vi "test Acyclic Loopback Selective Triggers.vi"(8 "error in":errorcluster, 11 "TestCase in":refnum<class "Single Board Loopback.lvclass">) -> (0 "error out":errorcluster, 3 "TestCase out":refnum<class "Single Board Loopback.lvclass">)   [LabVIEW 2020, in "Single Board Loopback.lvclass"]
uses:
  Single Board Loopback.lvclass
  C:/dev/git/niveristand-custom-device-testing-tools/VeriStandTestCase/VeriStandTestCase.lvclass
  <vilib>/numeric/Random Number (Range) U64.vi
  <vilib>/numeric/sub_Random U32.vi
  <vilib>/NI VeriStand/Execution/Workspace/NI VeriStand - Set Multiple Channel Values.vi
  <vilib>/addons/_JKI Toolkits/VI Tester/TestCase.llb/TestCase.lvclass
  <vilib>/NI VeriStand/Execution/Workspace/NI_VS Workspace ExecutionAPI.lvlib
  niveristand-custom-device-testing-tools/VeriStandTestUtilities/VeriStandTestUtilities.lvlib
  C:/Program Files (x86)/National Instruments/LabVIEW 2020/vi.lib/addons/_JKI Toolkits/VI Tester/TestCase.llb/TestCase.lvclass
  C:/dev/git/niveristand-aim-arinc429-custom-device/Source/Custom Device Support/Tests/System/Single Board Loopback/Single Board Loopback.lvclass
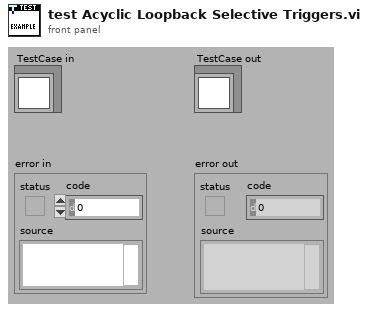
[diagram p1: front panel]
types:
  T1 = typedef "NI_VS Workspace ExecutionAPI.lvlib/WorkspaceAPI.ctl" = refnum<k24>
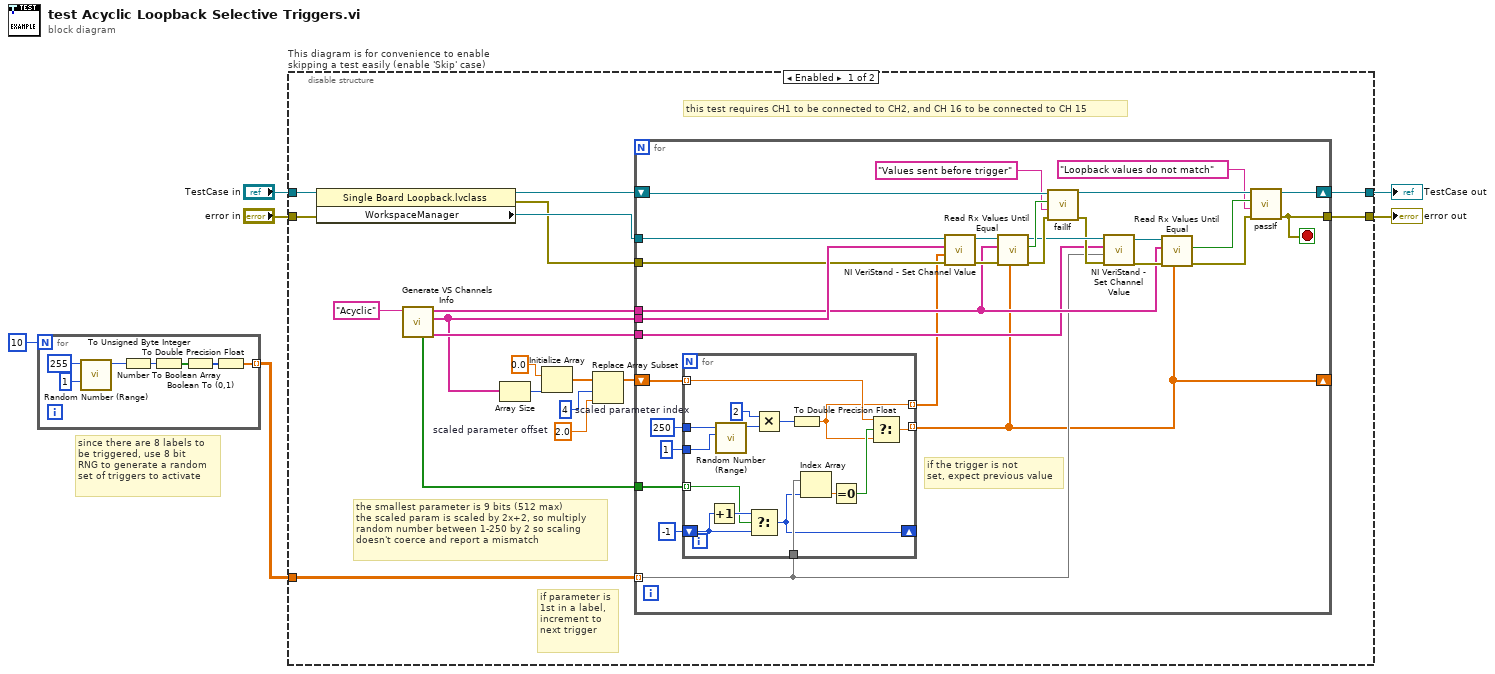
[diagram p0: block diagram]
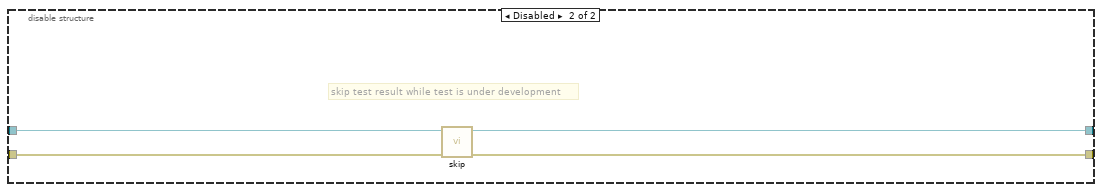
[diagram p2: hidden frame]
diagram:
  # "since there are 8 labels to\nbe triggered, use 8 bit \nRNG to generate a random\nset of triggers to activate"
  n1 = for {
    N: 10 -> [_]
    tunnel: [w7] -> w2 mode=indexing
    n2 = call-poly <vilib>:"Random Number (Range).vi"("lower bound (0)"=u64 1, "upper bound (100)"=u64 255) -> ("number"=w10:u64)  [unwired: 9 in]
    n3 = To Unsigned Byte Integer(number=w10) -> (unsigned 8bit integer=w9:u8)
    n4 = Number To Boolean Array(number=w9) -> (Boolean array=w13:bool[])
    n5 = Boolean To (0,1)(Boolean=w13) -> (0, 1=w8:i16[])
    n6 = To Double Precision Float(number=w8) -> (double precision float=w7:dbl[])
  }
  n7 = disable-structure "This diagram is for convenience to enable skipping a test easily (enable 'Skip' case)" shown="Enabled" {
    disable-tunnel: "TestCase in" -> [w28 w80]
    disable-tunnel: [w26 w78] -> w3
    disable-tunnel: [w25 w79] -> w5
    disable-tunnel: "error in" -> [w27 w77]
    disable-tunnel: w2 -> [w23 _]
    frame Enabled {
      w17 = 2.0  # scaled parameter offset
      w18 = 4  # scaled parameter index
      # "the smallest parameter is 9 bits (512 max)\nthe scaled param is scaled by 2x+2, so multiply \nrandom number between 1-250 by 2 so scaling\ndoesn't coerce and report a mismatch"
      # "if parameter is 1st in a label, increment to next trigger"
      # "this test requires CH1 to be connected to CH2, and CH 16 to be connected to CH 15"
      n8 = property class="Single Board Loopback.lvclass"(reference=w28, error in=w27) -> (reference out=w29:refnum<class "Single Board Loopback.lvclass">, error out=w30:errorcluster, "WorkspaceManager"=w31:T1)
      n9 = call "Generate VS Channels Info.vi"("Transfer Type"="Acyclic") -> ("Tx Trigger Channels Array"=w24:string[], "Tx Channels Array"=w16:string[], "Rx Channels Array"=w32:string[], "Is First Parameter? Array"=w14:bool[])  [unwired: 6 in, 1 out]
      n10 = Array Size(array=w16) -> (size(s)=w21:i32)
      n11 = Initialize Array(0.0 ("element"), w21) -> (w22:dbl[])
      n12 = Replace Array Subset(array=w22, new element=w17, index=w18) -> (w19:dbl[])
      n13 = for {
        tunnel: w32 -> [w47]
        tunnel: w31 -> [w59]
        tunnel: w30 -> [w52]
        tunnel: w16 -> [w58]
        shift-right: [w43] -> w26
        shift-left: w29 -> [w54]
        tunnel: [w42] -> w25
        tunnel: w24 -> [w39]
        tunnel: w23 -> [w38] mode=indexing
        shift-right: [w35] -> _
        shift-left: w19 -> [w36]
        tunnel: w14 -> [w33]
        stop <- w42 stop-if-true
        # "if the trigger is not\nset, expect previous value"
        n14 = for {
          tunnel: [w66] -> w35 mode=indexing
          tunnel: u64 250 ("upper bound (100)") -> [w75]
          tunnel: u64 1 ("upper bound (100)") -> [w74]
          tunnel: w38 -> [w71]
          shift-right: [w70] -> _
          shift-left: -1 -> [w68]
          tunnel: w36 -> [w64] mode=indexing
          tunnel: [w63] -> w34 mode=indexing
          tunnel: w33 -> [w62] mode=indexing
          n15 = Increment(x=w68) -> (x+1=w69:i32)
          n16 = call-poly <vilib>:"Random Number (Range).vi"("lower bound (0)"=w74, "upper bound (100)"=w75) -> ("number"=w76:u64)  [unwired: 9 in]
          n17 = Select(t=w69, s=w62, f=w68) -> (s? t:f=w70:i32)
          n18 = Multiply(x=u64 2, y=w76) -> (x*y=w73:u64)
          n19 = To Double Precision Float(number=w73) -> (double precision float=w63:dbl)
          n20 = Index Array(array=w71, index=w70) -> (element=w67:dbl)
          n21 = Equal To 0?(x=w67) -> (x = 0?=w65:bool)
          n22 = Select(t=w64, s=w65, f=w63) -> (s? t:f=w66:dbl)
        }
        n23 = call-poly <vilib>:"NI VeriStand - Set Channel Value.vi"("error in (no error)"=w52, "Values"=w34, "Channels"=w58, "WorkspaceManager in"=w59) -> ("error out"=w55:errorcluster, "WorkspaceManager out"=w57:T1)  [unwired: 6 in]
        n24 = call "Read Rx Values Until Equal.vi"("expected values"=w35, "error in"=w55, "Rx aliases"=w47, "workspace manager in"=w57) -> ("error out"=w56:errorcluster, "values equal expected"=w53:bool, "workspace manager out"=w51:T1)  [unwired: 5 in]
        n25 = call-dynamic "failIf.vi"("error in (no error)"=w56, "message (\"\")"="Values sent before trigger" ("message (\"\")"), "fail"=w53, "TestCase in"=w54) -> ("error out"=w50:errorcluster, "TestCase out"=w44:refnum<class "Single Board Loopback.lvclass">)  [unwired: 6 in]
        n26 = call-poly <vilib>:"NI VeriStand - Set Channel Value.vi"("error in (no error)"=w50, "Values"=w38, "Channels"=w39, "WorkspaceManager in"=w51) -> ("error out"=w48:errorcluster, "WorkspaceManager out"=w49:T1)  [unwired: 6 in]
        n27 = call "Read Rx Values Until Equal.vi"("expected values"=w35, "error in"=w48, "Rx aliases"=w47, "workspace manager in"=w49) -> ("error out"=w45:errorcluster, "values equal expected"=w46:bool)  [unwired: 5 in, 1 out]
        n28 = call-dynamic "passIf.vi"("error in (no error)"=w45, "message (\"\")"="Loopback values do not match" ("message (\"\")"), "pass"=w46, "TestCase in"=w44) -> ("error out"=w42:errorcluster, "TestCase out"=w43:refnum<class "Single Board Loopback.lvclass">)  [unwired: 6 in]
      }
    }
    frame Disabled {
      # "skip test result while test is under development"
      n29 = call <vilib>:"skip.vi"("error in (no error)"=w77, "TestCase in"=w80) -> ("error out"=w79:errorcluster, "TestCase out"=w78:refnum<class "Single Board Loopback.lvclass">)  [unwired: 8 in]
    }
  }
  "error out" <- w5
  "TestCase out" <- w3
